vi "Sensor de Flujo_HEGO_1.vi"() -> ()   [LabVIEW 2015]
uses:
  <vilib>/MakerHub/LINX/Public/Peripherals/Digital/Digital Read N Chans.vi
  <vilib>/MakerHub/LINX/Private/Local IO/LinxDigitalRead.vi
  <vilib>/MakerHub/LINX/Public/Utilities/Check Channel.vi
  <vilib>/MakerHub/LINX/Public/Utilities/Open Serial.vi
  <vilib>/MakerHub/LINX/Private/Utilties/Generate Error.vi
  <vilib>/ptbypt/NI_PtbyPt.lvlib
  <vilib>/MakerHub/LINX/LMH-LINX.lvlib
panel:
  out "Values":bool[](array[boolean])
  out "LITROS POR MINUTO SEN2":dbl
  in  "Digital I/O Pin (0) 2":u8
  in  "Digital I/O Pin (0)":u8
  in  "VISA resource":refnum<visa-resource-name>
  out "LITROS POR MINUTO":dbl(graph)
  out "Horizontal Graduated Bar":dbl(slide) scale=0.0..100.0
  out "LITROS POR MINUTO 2":dbl(knob) scale=0.0..100.0
  out "Numeric":i32
  out "PULSOS POR SEGUNDO":i32
  out "CONTRO TIEMPO":dbl
  out "CONTEO":i32
  out "?":bool
  out "LITROS POR MINUTO SEN1":dbl
  out "?":string
  out "?":bool
  in  "?":bool
  # "MEDICIÓN DE FLUJO ATRAVEZ DEL SENSOR YF-S201"
  # "Militros/min"
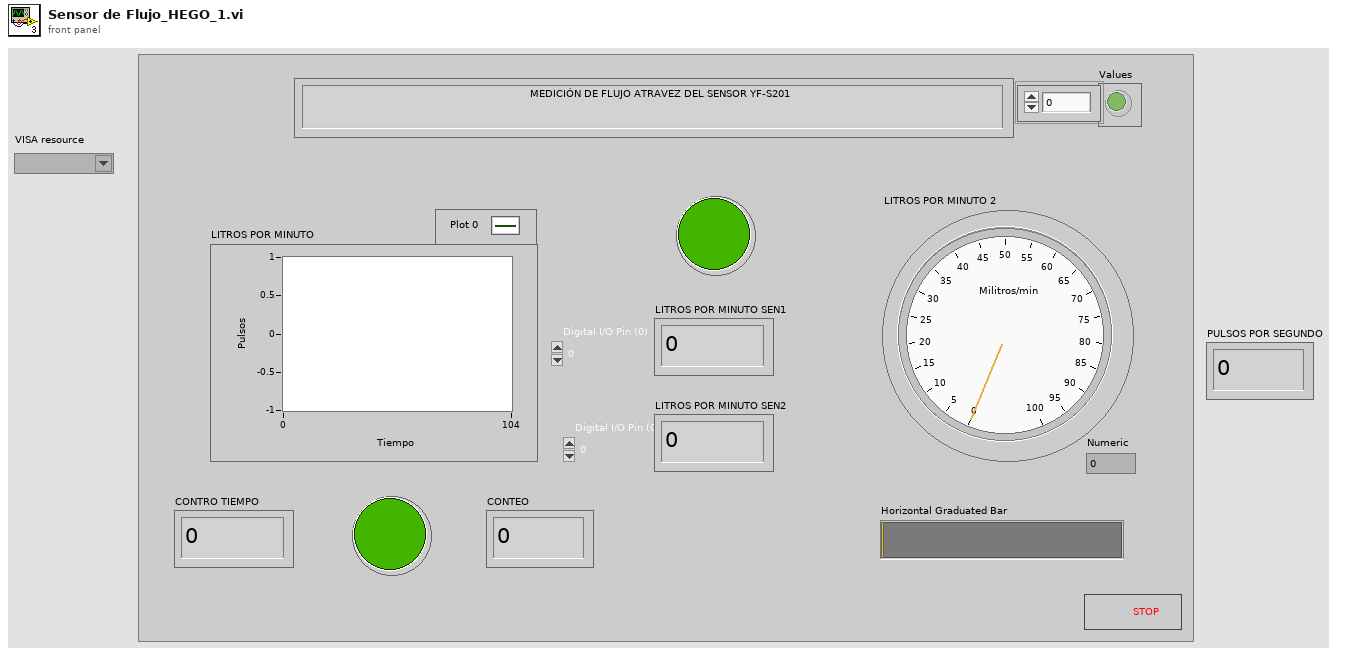
[diagram p1: front panel]
types:
  T1 = typedef "LMH-LINX.lvlib/LINX Ref.ctl" = cluster{"IO":T2, "Interface":T3, "LINX Device Config":T4}
  T2 = typedef "LMH-LINX.lvlib/Platform.ctl" = enum16{"Remote", "Local"}
  T3 = typedef "LMH-LINX.lvlib/Interface.ctl" = enum16{"Serial", "TCP"}
  T4 = typedef "LMH-LINX.lvlib/Device.lvlib/LINX Device Config.ctl" = cluster{"Interface":T3, "COM Port":refnum<visa-resource-name>, "TCP Configuration":T5, "Device Family":u8, "Device ID":u8, "Device Name":string, "TCP Ref":refnum<k5>, "Channels":T6}
  T5 = typedef "LMH-LINX.lvlib/Device.lvlib/TCP Config.ctl" = cluster{"IP Address":string, "Port":u16}
  T6 = typedef "LMH-LINX.lvlib/Channels.ctl" = cluster{"DI":u8[], "DO":u8[], "AI":u8[], "AO":u8[], "PWM":u8[], "QE":u8[], "UART":u8[], "I2C 2":u8[], "SPI":u8[], "CAN":u8[], "Servo":u8[], "AI Ref (V)":dbl, "AI Resolution (Bits)":u8, "AO Ref (V)":dbl, "AO Resolution (Bits)":u8}
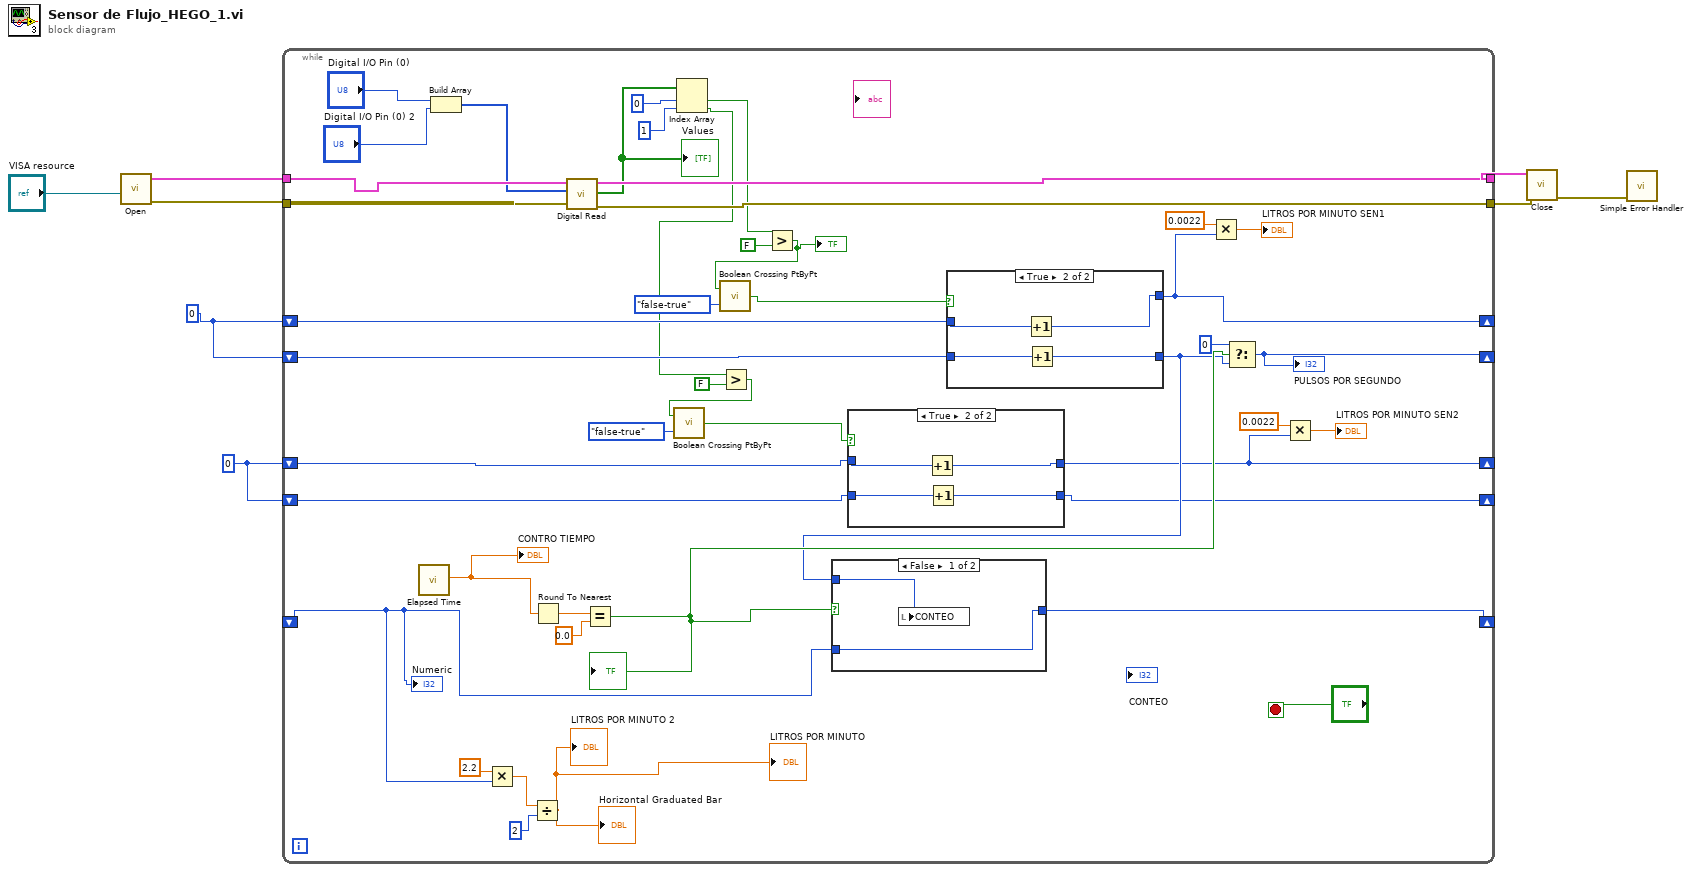
[diagram p0: block diagram]
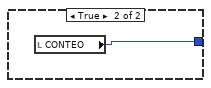
[diagram p3: hidden frame]
diagram:
  w1 = 0
  w2 = 0 ("CONTADOR 2")
  n1 = call-poly <vilib>:"Open.vi"("Serial Port"="VISA resource") -> ("Error Out"=w7:errorcluster, "LINX Resource"=w8:T1)  [unwired: 8 in, 1 out]
  n2 = while {
    tunnel: w8 -> [w30]
    tunnel: w7 -> [w29]
    tunnel: [w31] -> w5
    tunnel: [w28] -> w4
    shift-right: [w50] -> _
    shift-left: w2 -> [w49]
    shift-right: [w41] -> _
    shift-left: w2 -> [w45]
    shift-right: [w40] -> _
    shift-left: _ -> [w37]
    shift-right: [w9] -> _
    shift-left: w1 -> [w14]
    shift-right: [w13] -> _
    shift-left: w1 -> [w12]
    stop <- "?" stop-if-true
    n3 = call "Elapsed Time"() -> ("Elapsed Time (s)"=w35:dbl)  [unwired: 12 in, 7 out]
    "CONTRO TIEMPO" <- w35
    n4 = Build Array("Digital I/O Pin (0)", "Digital I/O Pin (0) 2") -> (w21:u8[])
    n5 = Multiply(x=2.2, y=w37) -> (x*y=w36:dbl)
    n6 = Divide(x=w36, y=2) -> (x/y=→"LITROS POR MINUTO 2" →"Horizontal Graduated Bar" →"LITROS POR MINUTO":dbl)
    n7 = Round To Nearest(number=w35) -> (nearest integer value=w34:dbl)
    n8 = call-poly <vilib>:"Digital Read.vi"("Error In"=w29, "DI Channels"=w21, "LINX Resource"=w30) -> ("Error Out"=w28:errorcluster, "Values"=w20:bool[], "LINX Resource"=w31:T1)  [unwired: 6 in]
    "Values" <- w20
    n9 = Equal?(x=w34, y=0.0) -> (x = y?=w43:bool)
    "?" <- w43
    n10 = Index Array(array=w20, index #1=0 ("index"), index #2=1 ("index")) -> (element #1=w17:bool, element #2=w16:bool)
    n11 = Greater?(x=w16, y=FALSE) -> (0:w26:bool)
    n12 = call <vilib>:"Boolean Crossing PtByPt.vi"("direction"=enum16{"either", "false-true", "true-false"}."false-true", "input"=w26) -> ("crossing"=w15:bool)  [unwired: 1 in]
    n13 = Greater?(x=w17, y=FALSE) -> (0:w24:bool)
    "?" <- w24
    n14 = call <vilib>:"Boolean Crossing PtByPt.vi"("direction"=enum16{"either", "false-true", "true-false"}."false-true", "input"=w24) -> ("crossing"=w47:bool)  [unwired: 1 in]
    n15 = case shown="True" w15 {
      tunnel: [w55 w59] -> w9
      tunnel: w14 -> [w55 w58]
      tunnel: w12 -> [w54 w57]
      tunnel: [w54 w56] -> w13
      frame False {
      }
      frame True {
        n16 = Increment(x=w58) -> (x+1=w59:i32)
        n17 = Increment(x=w57) -> (x+1=w56:i32)
      }
    }
    n18 = case shown="True" w47 {
      tunnel: [w64 w68] -> w50
      tunnel: w49 -> [w64 w67]
      tunnel: w45 -> [w63 w66]
      tunnel: [w63 w65] -> w42
      frame False {
      }
      frame True {
        n19 = Increment(x=w67) -> (x+1=w68:i32)
        n20 = Increment(x=w66) -> (x+1=w65:i32)
      }
    }
    n21 = case shown="False" w43 {
      tunnel: w42 -> [w61 _]
      tunnel: [w60 w62] -> w40
      tunnel: w37 -> [w60 _]
      frame False {
        n22 = local write "CONTEO"(w61) -> ()
      }
      frame True {
        n23 = local read "CONTEO"() -> (w62:i32)
      }
    }
    n24 = Multiply(x=0.0022, y=w50) -> (x*y=→"LITROS POR MINUTO SEN1":dbl)
    n25 = Select(t=0, s=w43, f=w42) -> (s? t:f=w41:i32)
    "PULSOS POR SEGUNDO" <- w41
    n26 = Multiply(x=0.0022, y=w9) -> (x*y=→"LITROS POR MINUTO SEN2":dbl)
    "Numeric" <- w37
  }
  n27 = call <vilib>:"Close.vi"("Error In"=w4, "LINX Resource"=w5) -> ("Error Out"=w3:errorcluster)  [unwired: 9 in]
  n28 = call <vilib>:"Simple Error Handler.vi"("error in (no error)"=w3) -> ()  [unwired: 4 in, 5 out]
